vi "Insert into Event Refnum Array.vi"(8 "error in (no error)":errorcluster, 11 "TwinCAT ADS in":refnum<class "TwinCAT ADS.lvclass">) -> (0 "error out":errorcluster, 3 "TwinCAT ADS out":refnum<class "TwinCAT ADS.lvclass">)   [LabVIEW 2018, in "TwinCAT ADS.lvclass"]
uses:
  TwinCAT ADS.lvclass
  TwinCAT ADS.lvclass/TwinCAT ADS.ctl
panel:
  in  "Event Callback":refnum<k27>
  in  "Event Registration Refnum":refnum<event-registration>
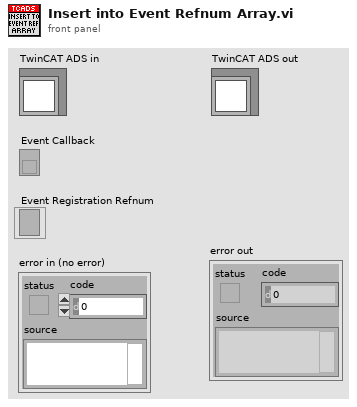
[diagram p1: front panel]
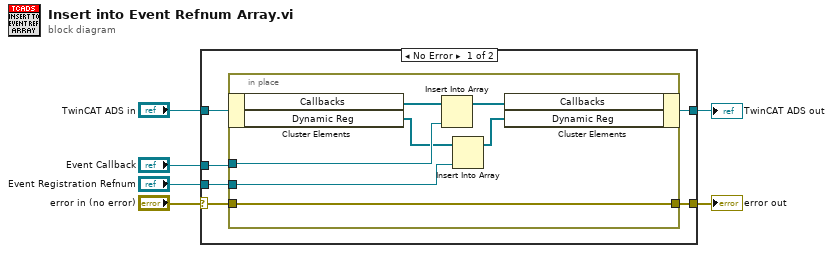
[diagram p0: block diagram]
diagram:
  n1 = case shown="No Error" "error in (no error)" {
    selector: "error in (no error)" -> [w7 w21]
    tunnel: "TwinCAT ADS in" -> [w12 w20]
    tunnel: "Event Registration Refnum" -> [w11 _]
    tunnel: [w10 w20] -> w3
    tunnel: [w9 w21] -> w4
    tunnel: "Event Callback" -> [w8 _]
    frame No Error {
      n2 = in-place {
        in-place-border: w8 -> [w17]
        in-place-border: [w19] -> w9
        in-place-border: w11 -> [w15]
        in-place-border: w7 -> [w19]
        n3 = in-place-cluster #1(w12) -> ("Callbacks"=w18:refnum<k27>[], "Dynamic Reg"=w14:refnum<event-registration>[])
        n4 = Insert Into Array(array=w18, new element=w17) -> (w16:refnum<k27>[])  [unwired: 1 in]
        n5 = Insert Into Array(array=w14, new element=w15) -> (w13:refnum<event-registration>[])  [unwired: 1 in]
        n6 = in-place-cluster #1("Callbacks"=w16, "Dynamic Reg"=w13) -> (w10:refnum<class "TwinCAT ADS.lvclass">)
      }
    }
    frame Error {
    }
  }
  "error out" <- w4
  "TwinCAT ADS out" <- w3
